vi "DMM Single Point Read.vi"() -> ()   [LabVIEW 2013]
uses:
  DMM/Signal Types.ctl
  Power Supply/AC Signal Data.ctl
  DMM.lvlib
  Power Supply.lvlib
  Fixture.lvlib
panel:
  in  "Serial Number":string="3"
  in  "DMM Channel":i32=1
  in  "outputVoltage":dbl=5.0 format="%#_13g"
  in  "PS channel":i32
  in  "AC Signal Data":T1={"Output Voltage"=14.0, "Frequency"=10.0, "Amplitude"=1.0}
  in  "signalType":T2
  out "error out":errorcluster
  out "Voltage":dbl
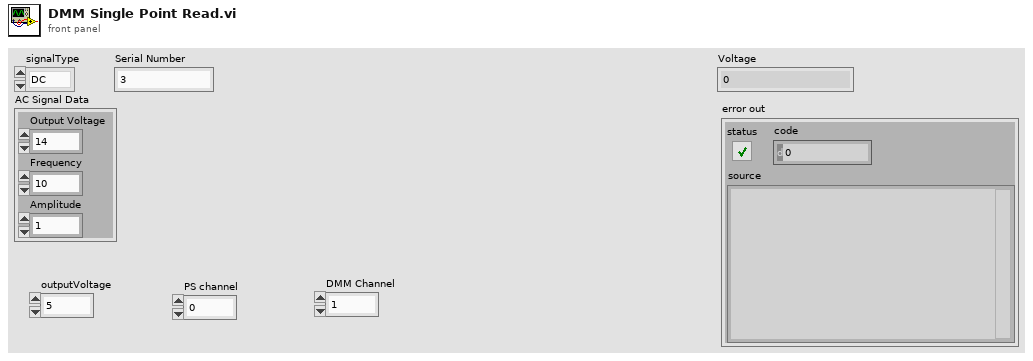
[diagram p1: front panel]
types:
  T1 = typedef "Driver Simulation.lvlib/Power Supply.lvlib/AC Signal Data.ctl" = cluster{"Output Voltage":dbl, "Frequency":dbl, "Amplitude":dbl}
  T2 = typedef "Driver Simulation.lvlib/DMM.lvlib/Signal Types.ctl" = enum16{"DC", "AC"}
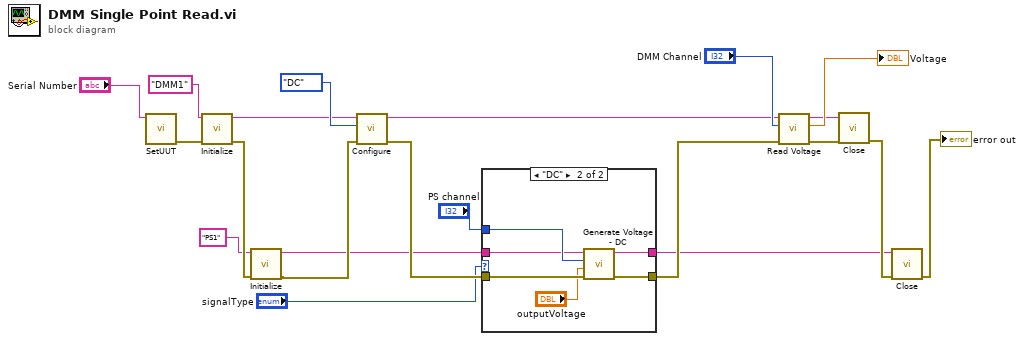
[diagram p0: block diagram]
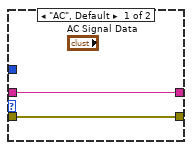
[diagram p2: hidden frame]
diagram:
  n1 = call "SetUUT.vi"("Serial Number"="Serial Number") -> ("error out"=w21:errorcluster)  [unwired: 10 in]
  n2 = call "Initialize.vi"("error in (no error)"=w21, "DMM in"="DMM1" ("Resource Name")) -> ("error out"=w20:errorcluster, "DMM out"=w1:string)  [unwired: 8 in]
  n3 = call "Initialize.vi"("error in (no error)"=w20, "Power Supply in"="PS1" ("Resource Name")) -> ("error out"=w8:errorcluster, "Power Supply out"=w5:string)  [unwired: 8 in]
  n4 = call "Configure.vi"("error in (no error)"=w8, "Signal Type"=Signal_Types."DC" ("signalType"), "DMM in"=w1) -> ("error out"=w18:errorcluster, "DMM out"=w3:string)  [unwired: 7 in]
  n5 = case shown="\"DC\"" "signalType" {
    tunnel: w18 -> [w22 w29]
    tunnel: [w22 w28] -> w10
    tunnel: [w23 w24] -> w7
    tunnel: "PS channel" -> [_ w27]
    tunnel: w5 -> [w23 w25]
    frame "AC", Default {
    }
    frame "DC" {
      n6 = call "Generate Voltage - DC.vi"("error in (no error)"=w29, "Output Voltage"="outputVoltage", "Channel"=w27, "Power Supply in"=w25) -> ("error out"=w28:errorcluster, "Power Supply out"=w24:string)  [unwired: 6 in]
    }
  }
  n7 = call "Read Voltage.vi"("error in (no error)"=w10, "Channel"="DMM Channel", "DMM in"=w3) -> ("error out"=w17:errorcluster, "Voltage"=→"Voltage":dbl, "DMM out"=w4:string)  [unwired: 6 in]
  n8 = call "Close.vi"("error in (no error)"=w17, "DMM in"=w4) -> ("error out"=w16:errorcluster)  [unwired: 9 in]
  n9 = call "Close.vi"("error in (no error)"=w16, "Power Supply in"=w7) -> ("error out"=→"error out":errorcluster)  [unwired: 9 in]
